vi "测试流程.vi"(11 "参数":T1) -> ()   [LabVIEW 2016]
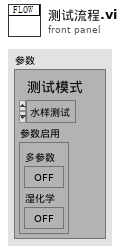
[diagram p1: front panel]
types:
  T1 = cluster{"测试模式":enum16{"水样测试", "平行样测试", "集成干预测试", "加标回收"}, "参数启用":cluster{"多参数":bool, "湿化学":bool}}
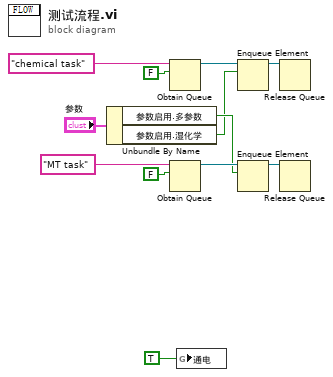
[diagram p0: block diagram]
diagram:
  n1 = Unbundle By Name("参数") -> ("参数启用.多参数"=w8:bool, "参数启用.湿化学"=w2:bool)
  n2 = Obtain Queue(name (unnamed)="chemical task" ("名称（未命名）"), element data type=FALSE) -> (queue out=w5:refnum<queue>)  [unwired: 3 in, 2 out]
  n3 = Obtain Queue(name (unnamed)="MT task" ("名称（未命名）"), element data type=FALSE) -> (queue out=w9:refnum<queue>)  [unwired: 3 in, 2 out]
  n4 = global write "系统设置全局变量.vi" "通电"(TRUE ("通电")) -> ()
  n5 = Enqueue Element(queue=w5, element=w2) -> (queue out=w6:refnum<queue>)  [unwired: 2 in, 2 out]
  n6 = Enqueue Element(queue=w9, element=w8) -> (queue out=w7:refnum<queue>)  [unwired: 2 in, 2 out]
  n7 = Release Queue(queue=w6) -> ()  [unwired: 2 in, 3 out]
  n8 = Release Queue(queue=w7) -> ()  [unwired: 2 in, 3 out]
